vi "TEST - Remove Msg Queue Element.vi"(8 "error in (no error)":errorcluster) -> (0 "error out":errorcluster, 2 "pass":bool)   [LabVIEW 2009]
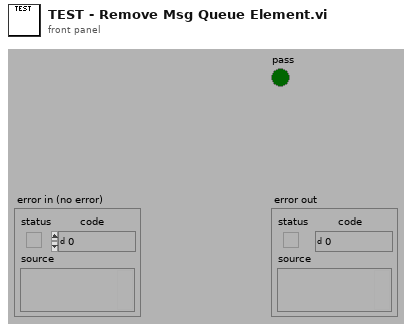
[diagram p1: front panel]
types:
  T1 = typedef "Msg Queue RefNum.ctl" = refnum<k1>
  T2 = typedef "Notifier RefNum" = refnum<k1>
  T3 = typedef "Msg Cluster.ctl" = cluster{"message":string, "response notifier":T2}
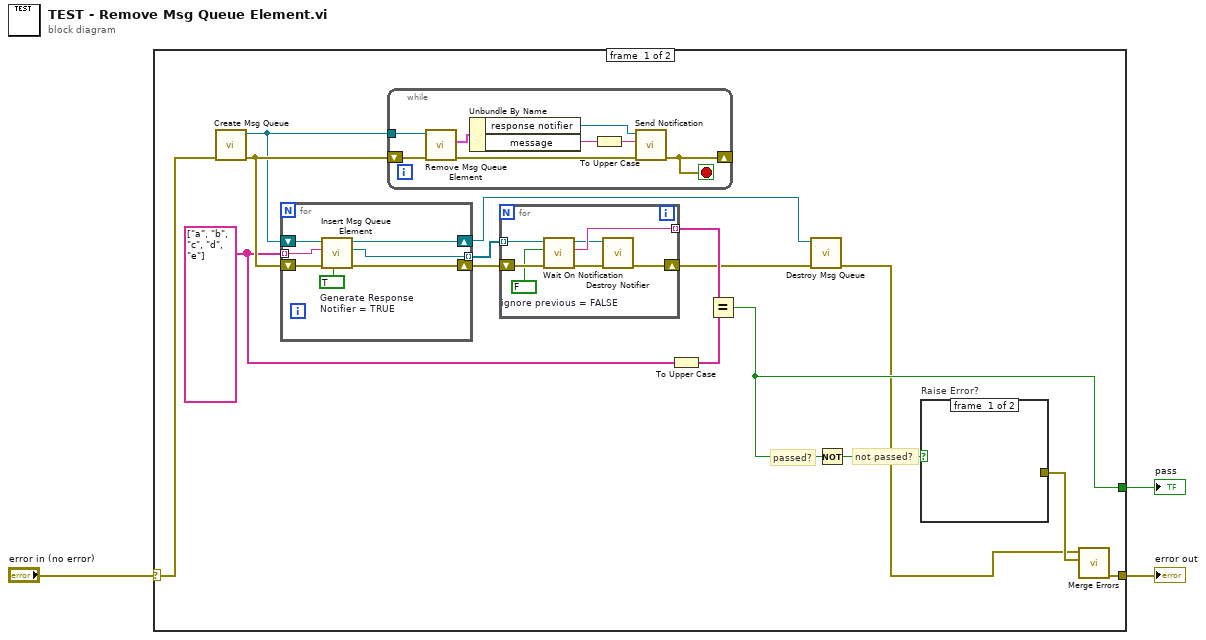
[diagram p0: block diagram]
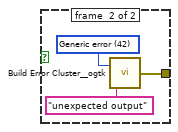
[diagram p2: hidden frame]
diagram:
  n1 = case shown="No Error" "error in (no error)" {
    selector: "error in (no error)" -> [w5 w44]
    tunnel: [w9 _] -> w3
    tunnel: [w18 w44] -> w1
    frame #0 {
      w12 = string[] ["a", "b", "c", "d", "e"]
      # "not passed?"
      # "passed?"
      n2 = call "Create Msg Queue.vi"("error in (no error)"=w5) -> ("error out"=w15:errorcluster, "msg queue"=w4:T1)  [unwired: 4 in, 1 out]
      n3 = for {
        tunnel: [w32] -> w14 mode=indexing
        tunnel: w12 -> [w31] mode=indexing
        shift-right: [w29] -> w7
        shift-left: w4 -> [w30]
        shift-right: [w27] -> w13
        shift-left: w15 -> [w28]
        w26 = TRUE  # Generate Response Notifier = TRUE
        n4 = call "Insert Msg Queue Element.vi"("Generate Response Notifier (F)"=w26, "error in (no error)"=w28, "message"=w31, "msg queue"=w30) -> ("error out"=w27:errorcluster, "response notifier"=w32:T2, "msg queue out"=w29:T1)  [unwired: 2 in, 1 out]
      }
      n5 = while {
        shift-right: [w33] -> _
        shift-left: w15 -> [w40]
        tunnel: w4 -> [w34]
        stop <- w33 stop-if-true
        n6 = call "Remove Msg Queue Element.vi"("error in (no error)"=w40, "msg queue"=w34) -> ("error out"=w35:errorcluster, "message"=w39:T3)  [unwired: 6 in, 2 out]
        n7 = Unbundle By Name(w39) -> ("response notifier"=w38:T2, "message"=w37:string)
        n8 = To Upper Case(1:w37) -> (0:w36:string)
        n9 = call <vilib>:"Send Notification.vi"("error in (no error)"=w35, "notification"=w36, "notifier"=w38) -> ("error out"=w33:errorcluster)  [unwired: 3 in, 1 out]
      }
      n10 = for {
        tunnel: w14 -> [w25] mode=indexing
        shift-right: [w20] -> w8
        shift-left: w13 -> [w24]
        tunnel: [w22] -> w11 mode=indexing
        w23 = FALSE  # ignore previous = FALSE
        n11 = call <vilib>:"Wait On Notification.vi"("error in (no error)"=w24, "ignore previous (T)"=w23, "notifier"=w25) -> ("error out"=w21:errorcluster, "notification"=w22:string, "notifier out"=w19:T2)  [unwired: 1 in, 1 out]
        n12 = call <vilib>:"Destroy Notifier.vi"("error in (no error)"=w21, "notifier"=w19) -> ("error out"=w20:errorcluster)  [unwired: 3 in, 2 out]
      }
      n13 = To Upper Case(1:w12) -> (0:w10:string[])
      n14 = Equal?(x=w11, y=w10) -> (x = y?=w9:bool)
      n15 = call "Destroy Msg Queue.vi"("error in (no error)"=w8, "msg queue"=w7) -> ("error out"=w6:errorcluster)  [unwired: 3 in, 2 out]
      n16 = Not(x=w9) -> (.not. x?=w16:bool)
      n17 = case "Raise Error?" shown="True" w16 {
        tunnel: [_ w41] -> w17
        frame #0 {
        }
        frame #1 {
          w42 = 42 items=["No error", "Argument error", "Memory is full", "Out of zone", "End of file", "File already open", "Generic file I/O error", "File not found", "File permission error", "Disk is full", "Duplicate path", "Too many files open", "System feature not enabled", "Resource file not found", "Cannot add resource", "Resource not found", "Image not found", "Image memory error", "Pen does not exist", "Config type invalid", "Config token not found", "Config parse error", "Config memory error", "Bad external code format", "Bad external code offset", "External code not present", "Null window", "Destroy window error", "Null menu", "Print aborted", "Bad print record", "Print driver error", "Windows error during printing", "Memory error during printing", "Print dialog error", "Generic print error", "Invalid device refnum", "Device not found", "Device parameter error", "Device unit error", "Cannot open device", "Device call aborted", "Generic error", "Cancelled by user", "Object ID too low", "Object ID too high", "Object not in heap", "Unknown heap", "Unknown object (invalid DefProc)", "Unknown object (DefProc not in table)", "Message out of range", "Invalid (null) method", "Unknown message", "Manager call not supported", "Bad address", "Network operation in progress", "Network operation timed out", "Connection is busy", "Network attribute not supported", "Network error", "Address in use", "System out of memory", "Connection aborted", "Connection refused", "Not connected", "Already connected", "Connection closed", "Initialization error (interapplication manager)", "Bad occurrence", "Wait on unbound occurrence handler", "Occurrence queue overflow", "Datalog type conflict", "Unused", "Unrecognized type (interapplication manager)", "Memory corrupt", "Failed to make temporary DLL", "Old CIN version", "Drag socket not found", "Failed to load drop-object", "Failed to register OLE object", "Failed to release OLE object", "Format specifier type mismatch", "Unknown format specifier", "Too few format specifiers", "Too many format specifiers", "Scan failed", "Newer CIN version", "Error converting to variant", "Runtime menu error", "Password tampered", "Variant attribute not found", "Incompatible variant data type", "Event data is not available", "Event Store is not present", "Occurrence is not found", "Event Queue is not created", "Event info is not available", "Refnum passed is NULL", "Error retrieving Class GUID", "Error retrieving CoClass GUID", "Error retrieving TypeLib GUID.", "Bad built application magic bytes.", "Specific driver is different from the specific driver associated with the Logical Name.", "There is no session opened to the class driver.", "Max Error", "MAX - Error with config objects", "MAX - Error loading configuration", "MAX - Group not supported"]
          n18 = call <userlib>:"Build Error Cluster__ogtk.vi"("String to Prepend to source (\"\")"="unexpected output" ("String to Prepend to source (\"\")"), "code"=w42) -> ("error out"=w41:errorcluster)
        }
      }
      n19 = call <vilib>:"Merge Errors.vi"("error in 2 (no error)"=w17, "error in 1 (no error)"=w6) -> ("error out"=w18:errorcluster)  [unwired: 5 in]
    }
    frame #1 {
    }
  }
  "pass" <- w3
  "error out" <- w1
